vi "_CSMObj-Release Chain Node.vi"(8 "Error In":errorcluster caption="error in (no error)", 11 "CSMQ In":T1={"info"={"Module Name"="", "Requested Name"="", "Group Name"="", "Mode"=enum."Stand Alone", "Allowed Messages"=[]}, "Refs"={"WatchDogQ"=refnum, "CSMDataDVR"=refnum, "Queue"={"HPriorityQ"=refnum, "LowPriorityQ"=refnum}, "GroupDataDVR"=refnum, "TagMap"=refnum, "ExitEvent"=refnum, "NewStateEvent"=refnum, "StatusEvent"=refnum, "InterruptEvent"=refnum}}) -> (0 "error out":errorcluster, 1 "Group Release?":bool, 3 "CSMQ Out":T1={"info"={"Module Name"="", "Requested Name"="", "Group Name"="", "Mode"=enum."Stand Alone", "Allowed Messages"=[]}, "Refs"={"WatchDogQ"=refnum, "CSMDataDVR"=refnum, "Queue"={"HPriorityQ"=refnum, "LowPriorityQ"=refnum}, "GroupDataDVR"=refnum, "TagMap"=refnum, "ExitEvent"=refnum, "NewStateEvent"=refnum, "StatusEvent"=refnum, "InterruptEvent"=refnum}})   [LabVIEW 2017, in "Communicable State Machine.lvlib"]
uses:
  Communicable State Machine.lvlib
  _CSMObj.ctl
  _CSMObj-Info.ctl
  Typedef/_CSM_MODE.ctl
  _CSMObj-Refs.ctl
  _CSMObj-Data.ctl
  Priority Queue/Priority Queue.ctl
  Typedef/_Cross CSM State Data.ctl
  Typedef/_CSM_MSG_TYPE.ctl
  Typedef/_Cross CSM State Response.ctl
  Typedef/_CSM_Response Source Message.ctl
  Priority Queue/def-Data(LowPRI-Q).ctl
  _CSMObj-ModeData.ctl
  Typedef/_CSM Status Change Event Data.ctl
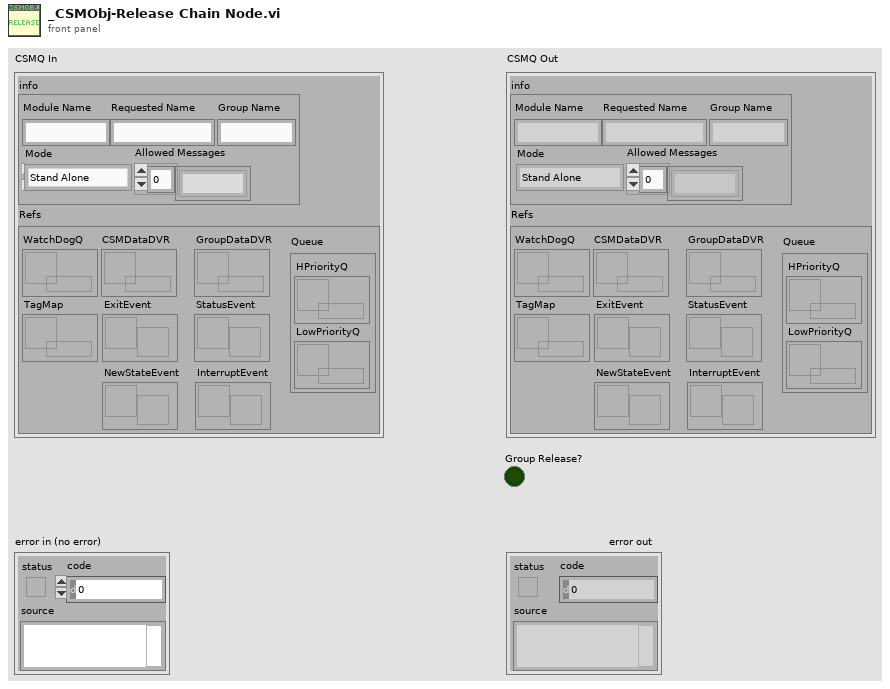
[diagram p1: front panel]
types:
  T1 = typedef "Communicable State Machine.lvlib/_CSMObj.ctl" = cluster{"info":T2, "Refs":T4}
  T2 = typedef "Communicable State Machine.lvlib/_CSMObj-Info.ctl" = cluster{"Module Name":string, "Requested Name":string, "Group Name":string, "Mode":T3, "Allowed Messages":string[]}
  T3 = typedef "Communicable State Machine.lvlib/_CSM_MODE.ctl" = enum16{"Not Exist", "Stand Alone", "CSM", "Worker", "Worker Agent", "Chain Node", "Chain"}
  T4 = typedef "Communicable State Machine.lvlib/_CSMObj-Refs.ctl" = cluster{"WatchDogQ":refnum<queue>, "CSMDataDVR":refnum<data-value>, "Queue":T5, "GroupDataDVR":refnum<data-value>, "TagMap":refnum<data-value>, "ExitEvent":refnum<user-event>, "NewStateEvent":refnum<user-event>, "StatusEvent":refnum<user-event>, "InterruptEvent":refnum<user-event>}
  T5 = typedef "Communicable State Machine.lvlib/Priority Queue.ctl" = cluster{"HPriorityQ":refnum<queue>, "LowPriorityQ":refnum<queue>}
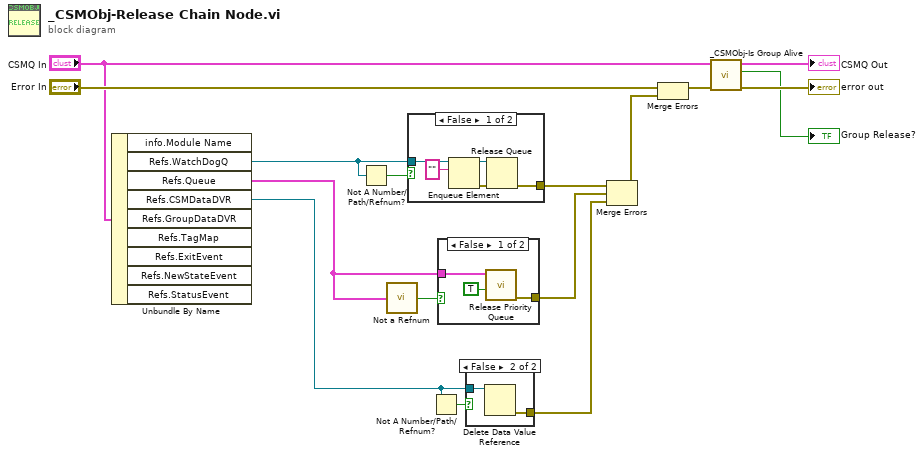
[diagram p0: block diagram]
diagram:
  n1 = Unbundle By Name("CSMQ In") -> ("Refs.WatchDogQ"=w11:refnum<queue>, "Refs.Queue"=w6:T5, "Refs.CSMDataDVR"=w9:refnum<data-value>)  [unwired: 6 out]
  n2 = Not A Number/Path/Refnum?(number/path/refnum=w11) -> (NaN/Path/Refnum?=w12:bool)
  n3 = call "Not a Refnum.vi"("Priority Queue.lvclass"=w6) -> ("NaN/Path/Refnum?"=w8:bool)  [unwired: 4 in]
  n4 = case shown="False" w12 {
    tunnel: [w21 _] -> w10
    tunnel: w11 -> [w20 _]
    frame False {
      n5 = Enqueue Element(queue=w20, element="") -> (queue out=w19:refnum<queue>, error out=w17:errorcluster)  [unwired: 2 in, 1 out]
      n6 = Release Queue(queue=w19, error in (no error)=w17) -> (error out=w21:errorcluster)  [unwired: 1 in, 2 out]
    }
    frame True {
    }
  }
  n7 = Not A Number/Path/Refnum?(number/path/refnum=w9) -> (NaN/Path/Refnum?=w13:bool)
  n8 = case shown="False" w8 {
    tunnel: w6 -> [w24 _]
    tunnel: [w22 _] -> w7
    frame False {
      n9 = call "Release Priority Queue.vi"("Force Destroy? (F)"=TRUE ("force destroy? (F)"), "Priority Queue"=w24) -> ("error out"=w22:errorcluster)  [unwired: 9 in]
    }
    frame True {
    }
  }
  n10 = case shown="False" w13 {
    tunnel: [_ w26] -> w14
    tunnel: w9 -> [_ w25]
    frame True {
    }
    frame False {
      n11 = Delete Data Value Reference(data value reference=w25) -> (error out=w26:errorcluster)  [unwired: 1 in, 1 out]
    }
  }
  n12 = Merge Errors(w10, w7, w14) -> (w15:errorcluster)
  n13 = Merge Errors("Error In", w15) -> (w5:errorcluster)
  n14 = call "_CSMObj-Is Group Alive.vi"("error in (no error)"=w5, "CSMQ In"="CSMQ In") -> ("error out"=→"error out":errorcluster, "Group Alive?"=→"Group Release?":bool, "CSMQ Out"=→"CSMQ Out":T1)  [unwired: 7 in]
